vi "Configure Bitfile.vi"(0 "USRP RIO device":T1, 1 "Rx?":bool, 5 "which bitfile":string(combo)="Time", 11 "error in":errorcluster) -> (4 "USRP RIO device":T1, 6 "bitfile":path, 15 "error out":errorcluster)   [LabVIEW 2016]
uses:
  <vilib>/userdefined/Silver/nirio_resource_slv.ctl
  <vilib>/Utility/error.llb/Error Cluster From Error Code.vi
  <vilib>/regexp/Match Regular Expression.xnode
  <vilib>/ErrorRing/Error Ring.xnode
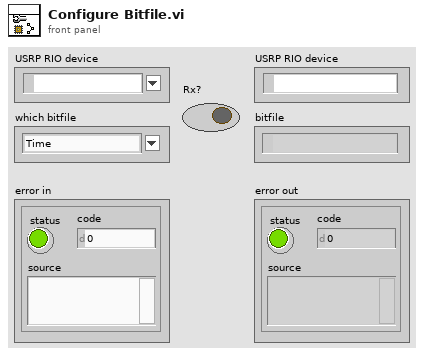
[diagram p1: front panel]
types:
  T1 = typedef "nirio_resource_slv.ctl" = tag
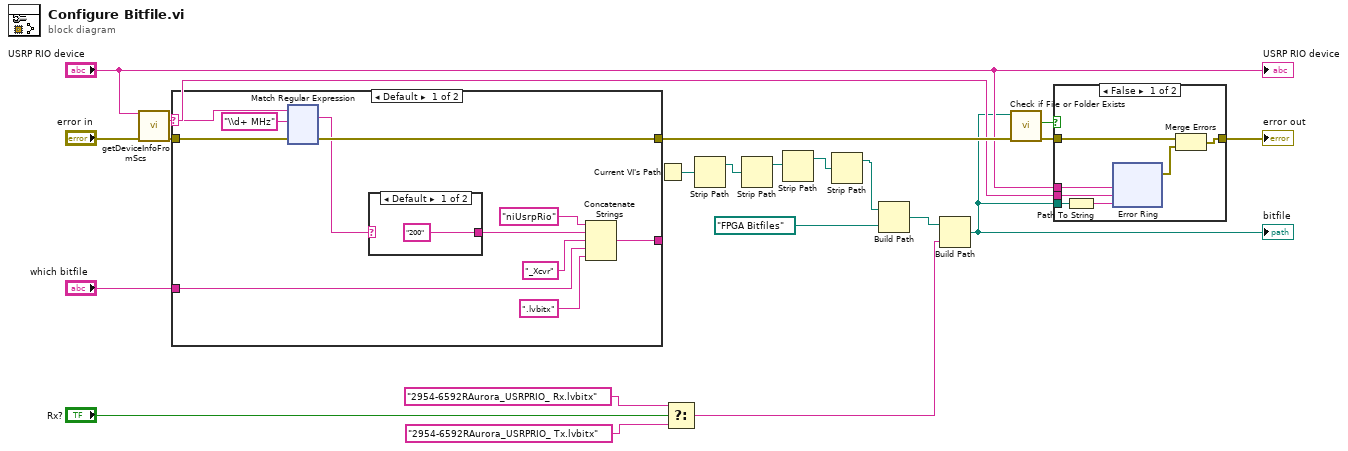
[diagram p0: block diagram]
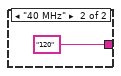
[diagram p3: hidden frame]
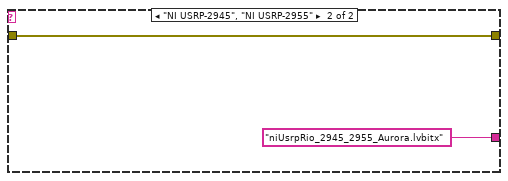
[diagram p4: hidden frame]
diagram:
  n1 = call <vilib>:"getDeviceInfoFromScs.vi"("rio device"="USRP RIO device", "error in"="error in") -> ("product name"=w12:string, "error out"=w14:errorcluster)  [unwired: 9 in, 3 out]
  n2 = case shown="Default" w12 {
    selector: w12 -> [w22 _]
    tunnel: "which bitfile" -> [w29 _]
    tunnel: w14 -> [w27 w149]
    tunnel: [w26 w149] -> w13
    tunnel: [w23 "niUsrpRio_2945_2955_Aurora.lvbitx" ("f")] -> _
    frame Default {
      n3 = xnode "Match Regular Expression"("input string"=w22, "regular expression"="\\d+ MHz", "error in"=w27) -> ("whole match"=w25:string, "error out"=w26:errorcluster)  [unwired: 3 in, 3 out]
      n4 = case shown="Default" w25 {
        tunnel: ["200" ("format string") "120" ("format string")] -> w24
        frame Default {
        }
        frame "40 MHz" {
        }
      }
      n5 = Concatenate Strings("niUsrpRio" ("format string"), w24, "_Xcvr" ("format string"), w29, ".lvbitx" ("format string")) -> (w23:string)
    }
    frame "NI USRP-2945", "NI USRP-2955" {
    }
  }
  n6 = Current VI's Path() -> (path=w21:path)
  n7 = Select(t="2954-6592RAurora_USRPRIO_ Rx.lvbitx" ("format string"), s="Rx?", f="2954-6592RAurora_USRPRIO_ Tx.lvbitx" ("format string")) -> (s? t:f=w2:string)
  n8 = Strip Path(path=w21) -> (stripped path=w18:path)  [unwired: 1 out]
  n9 = Strip Path(path=w18) -> (stripped path=w17:path)  [unwired: 1 out]
  n10 = Strip Path(path=w17) -> (stripped path=w7:path)  [unwired: 1 out]
  n11 = Strip Path(path=w7) -> (stripped path=w6:path)  [unwired: 1 out]
  n12 = Build Path(base path=w6, name or relative path=path "FPGA Bitfiles") -> (appended path=w19:path)
  n13 = Build Path(base path=w19, name or relative path=w2) -> (appended path=w1:path)
  "bitfile" <- w1
  n14 = call <vilib>:"Check if File or Folder Exists.vi"("error in (no error)"=w13, "path"=w1) -> ("error out"=w9:errorcluster, "file or folder exists?"=w8:bool)  [unwired: 7 in, 1 out]
  n15 = case shown="False" w8 {
    tunnel: w1 -> [w157 _]
    tunnel: w12 -> [w155 _]
    tunnel: "USRP RIO device" -> [w154 _]
    tunnel: [w152 w167] -> w10
    tunnel: w9 -> [w153 w167]
    frame False {
      n16 = Path To String(path=w157) -> (string=w156:string)
      n17 = xnode "Error Ring"("parameter 0"=w154, "parameter 1"=w155, "parameter 2"=w156) -> ("error out"=w151:errorcluster)
      n18 = Merge Errors(w153, w151) -> (w152:errorcluster)
    }
    frame True {
    }
  }
  "error out" <- w10
  "USRP RIO device" <- "USRP RIO device"
